vi "ChoreoLoadTrajectory.vi"(11 "trajectoryJsonString":string) -> (0 "Error":bool, 1 "Samples":T1(array[cluster]), 2 "sampleType":string, 3 "ChoreoTrajectorySwerve":T2)   [LabVIEW 2025]
doc: "Parse a Swerve choreo trajectory from a JSON formatted string. \n\nInputs: \n - trajectoryJsonString - string- The string containing the choreo trajectory. Note that files may have a .TRAJ extension. These are actually internally formatted as JSON files.\n\nOutputs:\n - ChoreoTrajectorySwerve - cluster - Trajectory read from JSON file.\n - Error - boolean - TRUE if an error occured."
uses:
  <vilib>/Rock Robotics/WPI/ThirdParty/ChoreoLib/TypeDef/ChoreoEventMarker.ctl
  <vilib>/Rock Robotics/WPI/ThirdParty/ChoreoLib/TypeDef/ChoreoTrajectorySwerve.ctl
  <vilib>/Rock Robotics/WPI/ThirdParty/ChoreoLib/TypeDef/ChoreoSwerveSample.ctl
  <vilib>/Rock Robotics/WPI/ThirdParty/ChoreoLib/ChoreoLib.lvlib
panel:
  out "nameErr":bool
  out "EventsEmpty":bool
  out "EventMarkers":T4[](array[typedef])
  out "splitsErr":bool
  out "version":i32
  out "VersionErr":bool
  out "SampleTypeErr":bool
  in  "?":T1(array[cluster])
  out "sampleError":bool
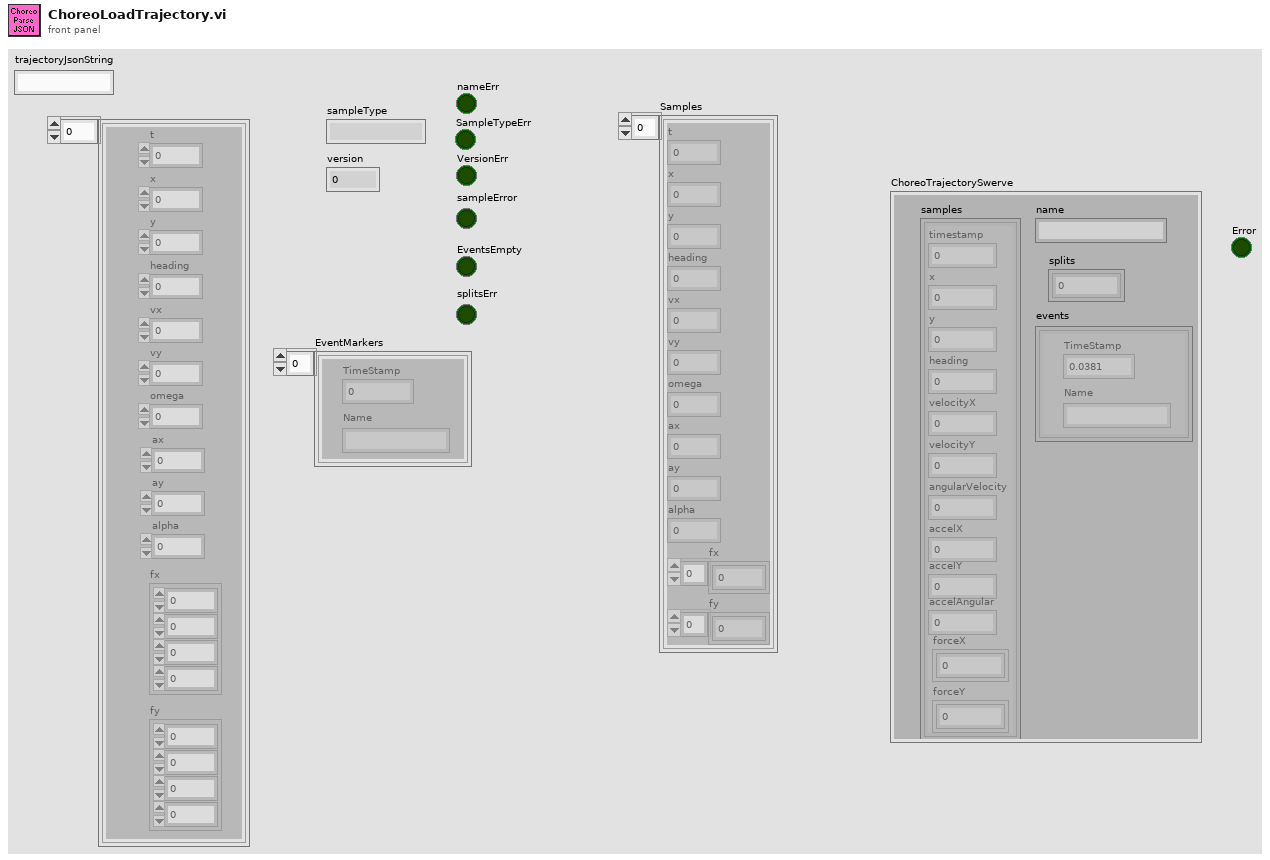
[diagram p1: front panel]
types:
  T1 = cluster{"t":dbl, "x":dbl, "y":dbl, "heading":dbl, "vx":dbl, "vy":dbl, "omega":dbl, "ax":dbl, "ay":dbl, "alpha":dbl, "fx":dbl[], "fy":dbl[]}[]
  T2 = typedef "ChoreoLib.lvlib/ChoreoTrajectorySwerve.ctl" = cluster{"name":string, "samples":T3[], "splits":i32[], "events":T4[]}
  T3 = typedef "ChoreoLib.lvlib/ChoreoSwerveSample.ctl" = cluster{"timestamp":dbl, "x":dbl, "y":dbl, "heading":dbl, "velocityX":dbl, "velocityY":dbl, "angularVelocity":dbl, "accelX":dbl, "accelY":dbl, "accelAngular":dbl, "forceX":dbl[], "forceY":dbl[]}
  T4 = typedef "ChoreoLib.lvlib/ChoreoEventMarker.ctl" = cluster{"TimeStamp":dbl, "Name":string}
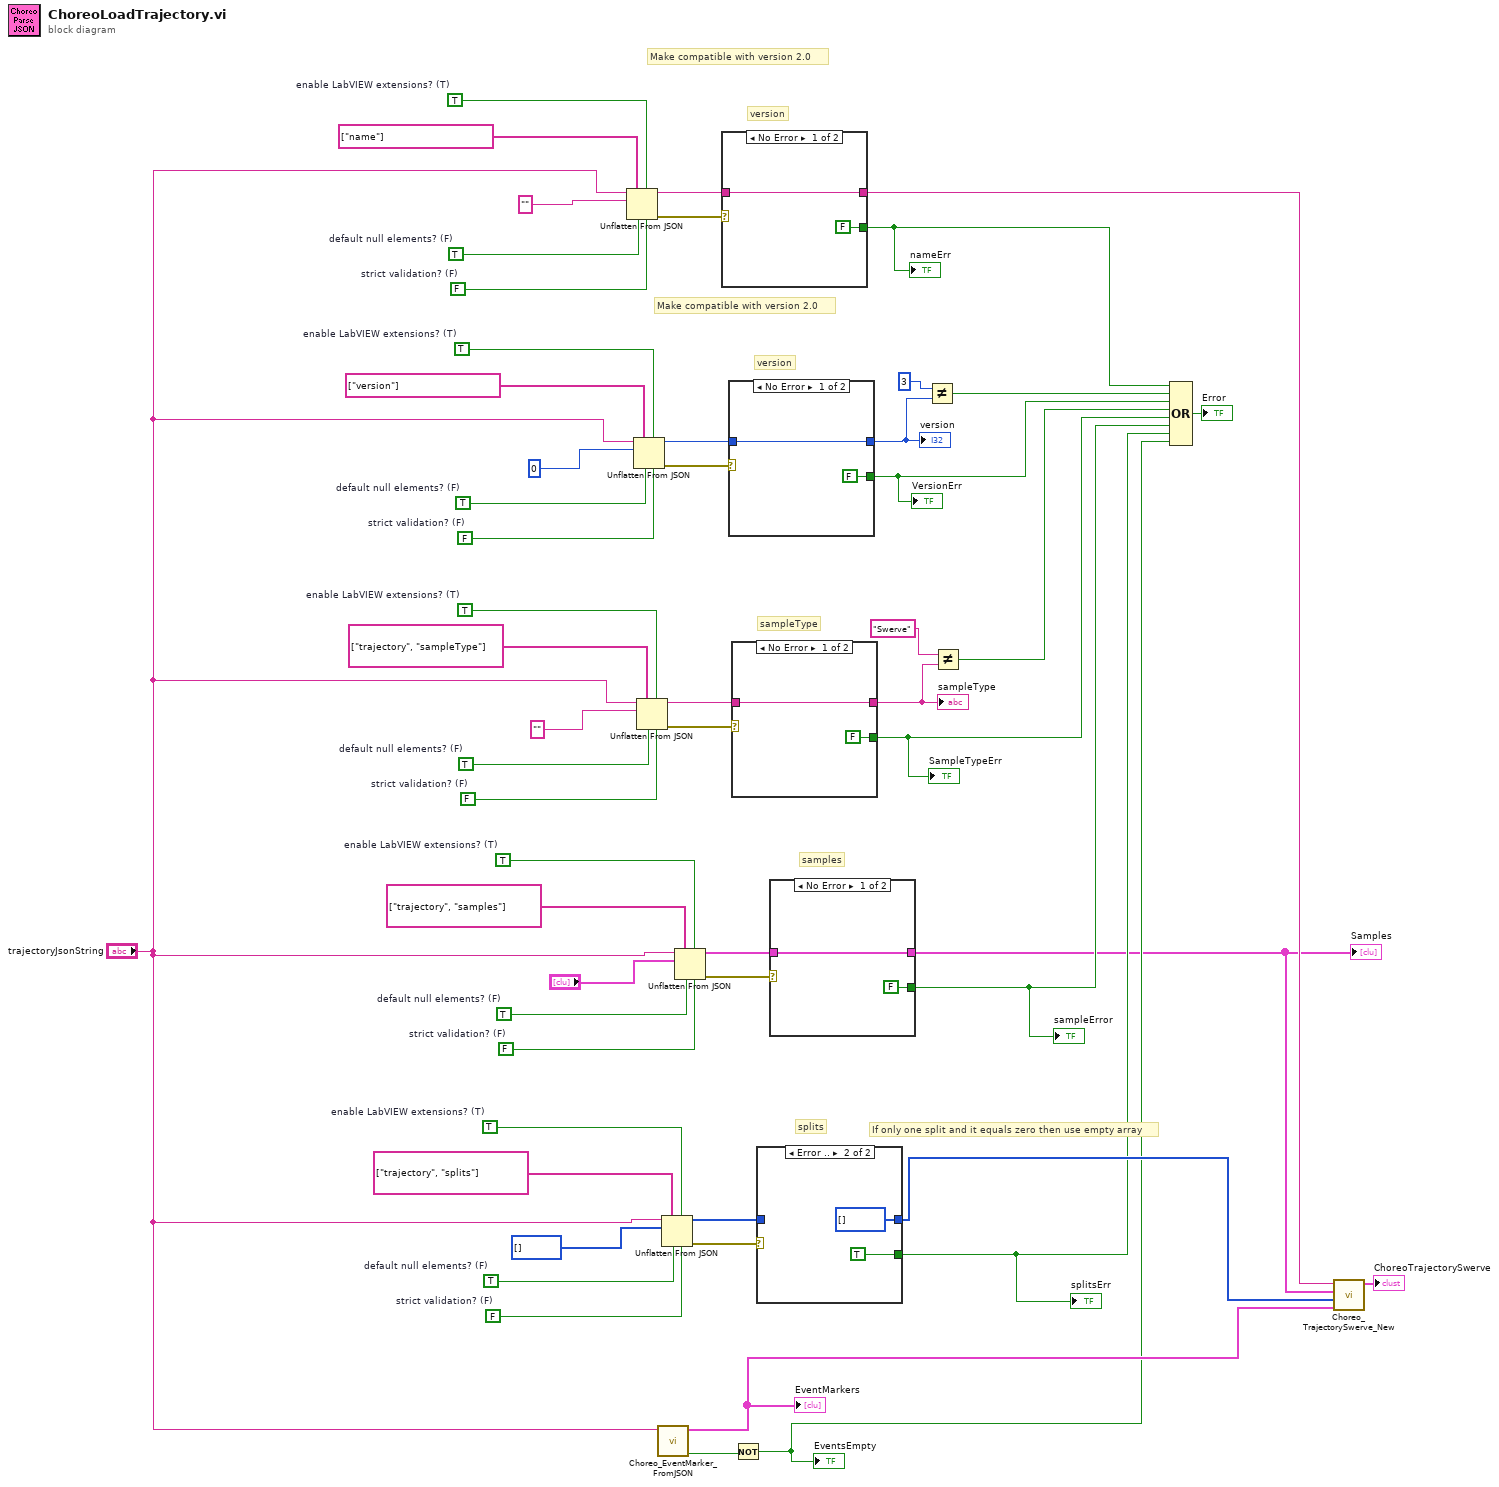
[diagram p0: block diagram]
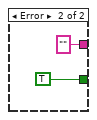
[diagram p2: hidden frame]
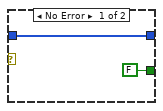
[diagram p3: hidden frame]
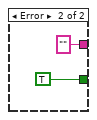
[diagram p4: hidden frame]
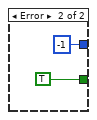
[diagram p5: hidden frame]
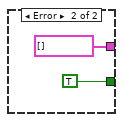
[diagram p6: hidden frame]
diagram:
  w21 = FALSE  # strict validation? (F)
  w22 = TRUE  # default null elements? (F)
  w23 = TRUE  # enable LabVIEW extensions? (T)
  w30 = FALSE  # strict validation? (F)
  w31 = TRUE  # default null elements? (F)
  w32 = TRUE  # enable LabVIEW extensions? (T)
  w37 = FALSE  # strict validation? (F)
  w38 = TRUE  # default null elements? (F)
  w39 = TRUE  # enable LabVIEW extensions? (T)
  w44 = FALSE  # strict validation? (F)
  w45 = TRUE  # default null elements? (F)
  w46 = TRUE  # enable LabVIEW extensions? (T)
  w51 = FALSE  # strict validation? (F)
  w52 = TRUE  # default null elements? (F)
  w53 = TRUE  # enable LabVIEW extensions? (T)
  # "version"
  # "Make compatible with version 2.0"
  # "If only one split and it equals zero then use empty array"
  # "splits"
  # "samples"
  # "sampleType"
  # "version"
  # "Make compatible with version 2.0"
  n1 = Unflatten From JSON(path=string[] ["name"] ("path 7"), enable LabVIEW extensions? (T)=w23, JSON string="trajectoryJsonString", type and defaults="", default null elements? (F)=w22, strict validation? (F)=w21) -> (value=w24:string, error out=w25:errorcluster)  [unwired: 1 in]
  n2 = Unflatten From JSON(path=string[] ["version"] ("path 7"), enable LabVIEW extensions? (T)=w46, JSON string="trajectoryJsonString", type and defaults=0, default null elements? (F)=w45, strict validation? (F)=w44) -> (value=w47:i32, error out=w48:errorcluster)  [unwired: 1 in]
  n3 = Unflatten From JSON(path=string[] ["trajectory", "sampleType"] ("path 7"), enable LabVIEW extensions? (T)=w39, JSON string="trajectoryJsonString", type and defaults="", default null elements? (F)=w38, strict validation? (F)=w37) -> (value=w40:string, error out=w41:errorcluster)  [unwired: 1 in]
  n4 = call <vilib>:"Choreo_EventMarker_FromJSON.vi"("JSON String"="trajectoryJsonString") -> ("Exists"=w27:bool, "EventMarkers"=w6:T4[])  [unwired: 9 in]
  "EventMarkers" <- w6
  n5 = Unflatten From JSON(path=string[] ["trajectory", "splits"] ("path 7"), enable LabVIEW extensions? (T)=w32, JSON string="trajectoryJsonString", type and defaults=i32[] [], default null elements? (F)=w31, strict validation? (F)=w30) -> (value=w33:i32[], error out=w34:errorcluster)  [unwired: 1 in]
  n6 = Unflatten From JSON(path=string[] ["trajectory", "samples"] ("path 7"), enable LabVIEW extensions? (T)=w53, JSON string="trajectoryJsonString", type and defaults="?", default null elements? (F)=w52, strict validation? (F)=w51) -> (value=w54:T1, error out=w55:errorcluster)  [unwired: 1 in]
  n7 = case shown="No Error" w25 {
    tunnel: w24 -> [w56 _]
    tunnel: [FALSE TRUE] -> w16
    tunnel: [w56 ""] -> w17
    frame No Error {
    }
    frame Error {
    }
  }
  "nameErr" <- w16
  n8 = case shown="No Error" w48 {
    tunnel: w47 -> [w60 _]
    tunnel: [FALSE TRUE] -> w12
    tunnel: [w60 -1] -> w15
    frame No Error {
    }
    frame Error {
    }
  }
  "VersionErr" <- w12
  "version" <- w15
  n9 = case shown="No Error" w41 {
    tunnel: w40 -> [w64 _]
    tunnel: [FALSE TRUE] -> w8
    tunnel: [w64 ""] -> w11
    frame No Error {
    }
    frame Error {
    }
  }
  "SampleTypeErr" <- w8
  "sampleType" <- w11
  n10 = Not(x=w27) -> (.not. x?=w4:bool)
  "EventsEmpty" <- w4
  n11 = case shown="Error .." w34 {
    tunnel: w33 -> [w68 _]
    tunnel: [FALSE TRUE] -> w5
    tunnel: [w68 i32[] []] -> w26
    frame No Error {
    }
    frame Error {
    }
  }
  "splitsErr" <- w5
  n12 = case shown="No Error" w55 {
    tunnel: w54 -> [w72 _]
    tunnel: [FALSE TRUE] -> w7
    tunnel: [w72 T1 []] -> w1
    frame No Error {
    }
    frame Error {
    }
  }
  "sampleError" <- w7
  "Samples" <- w1
  n13 = Not Equal?(x=3, y=w15) -> (x != y?=w13:bool)
  n14 = Not Equal?(x="Swerve", y=w11) -> (x != y?=w9:bool)
  n15 = Compound Arithmetic op=OR(w16, w13, w12, w9, w8, w7, w5, w4) -> (→"Error":bool)
  n16 = call <vilib>:"Choreo_TrajectorySwerve_New.vi"("events"=w6, "splits"=w26, "samples"=w1, "name"=w17) -> ("ChoreoTrajectorySwerve"=→"ChoreoTrajectorySwerve":T2)  [unwired: 7 in]
